vi "BroadcastData.vi"(8 "error in (no error)":errorcluster, 10 "DataExchange":T1, 11 "DataProcessor in":refnum<class "DataProcessor.lvclass">) -> (0 "error out":errorcluster, 3 "DataProcessor out":refnum<class "DataProcessor.lvclass">)   [LabVIEW 2020, in "DataProcessor.lvlib" / "DataProcessor.lvclass"]
uses:
  DataProcessor.lvclass
  Hardware Abstraction Layer/Component/Device/Device/DataExchange.ctl
  DataProcessor.lvclass/DataProcessor.ctl
  Interface/DataListener Messages/OnDataChange Msg/OnDataChange Msg.lvclass/OnDataChange Msg.ctl
  <vilib>/ActorFramework/Message Enqueuer/Message Enqueuer.lvclass/Message Enqueuer.ctl
  <vilib>/ActorFramework/Message Enqueuer/Enqueue.vi
  Interface/DataListener Messages/OnDataChange Msg/OnDataChange Msg.lvclass
  C:/Program Files/National Instruments/LabVIEW 2020/vi.lib/ActorFramework/Message/Message.lvclass
  <vilib>/ActorFramework/Message Priority Queue/Priority Enqueue.vi
  Interface/DataListener/DataListener.lvclass
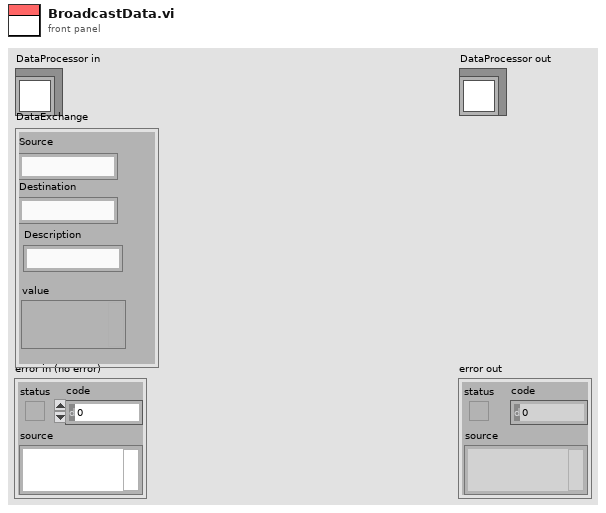
[diagram p1: front panel]
types:
  T1 = typedef "DataListener.lvclass/DataExchange.ctl" = cluster{"Source":string, "Destination":string, "Description":string, "value":variant}
  T2 = map{string, refnum<class "Message Enqueuer.lvclass">}
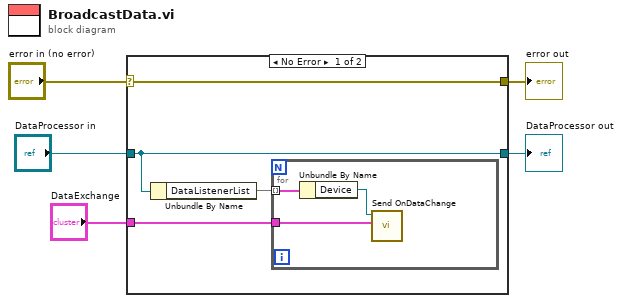
[diagram p0: block diagram]
diagram:
  n1 = case shown="No Error" "error in (no error)" {
    selector: "error in (no error)" -> [w6 w14]
    tunnel: [w6 w14] -> w1
    tunnel: [w9 w13] -> w2
    tunnel: "DataProcessor in" -> [w9 w13]
    tunnel: "DataExchange" -> [w7 _]
    frame No Error {
      n2 = Unbundle By Name(w9) -> ("DataListenerList"=w8:T2)
      n3 = for {
        tunnel: w8 -> [w12] mode=indexing
        tunnel: w7 -> [w10]
        n4 = Unbundle By Name(w12) -> ("Device"=w11:refnum<class "Message Enqueuer.lvclass">)
        n5 = call "Send OnDataChange.vi"("DataExchange"=w10, "Message Enqueuer"=w11) -> ()  [unwired: 8 in, 2 out]
      }
    }
    frame Error {
    }
  }
  "error out" <- w1
  "DataProcessor out" <- w2
